vi "LoggerHelper-Pnumatics.vi"(8 "Stablizer":T1, 9 "Grabber":T1, 10 "Intake":T1, 11 "Shifter":T1) -> (2 "Logged PNU Output":string)   [LabVIEW 2014]
uses:
  <vilib>/Rock Robotics/WPI/Solenoid/WPI_SolenoidValue.ctl
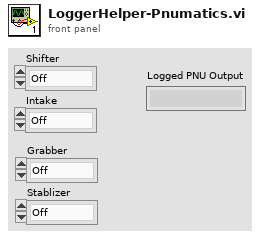
[diagram p1: front panel]
types:
  T1 = typedef "WPI_SolenoidValue.ctl" = enum16{"Off", "On", "Forward", "Reverse"}
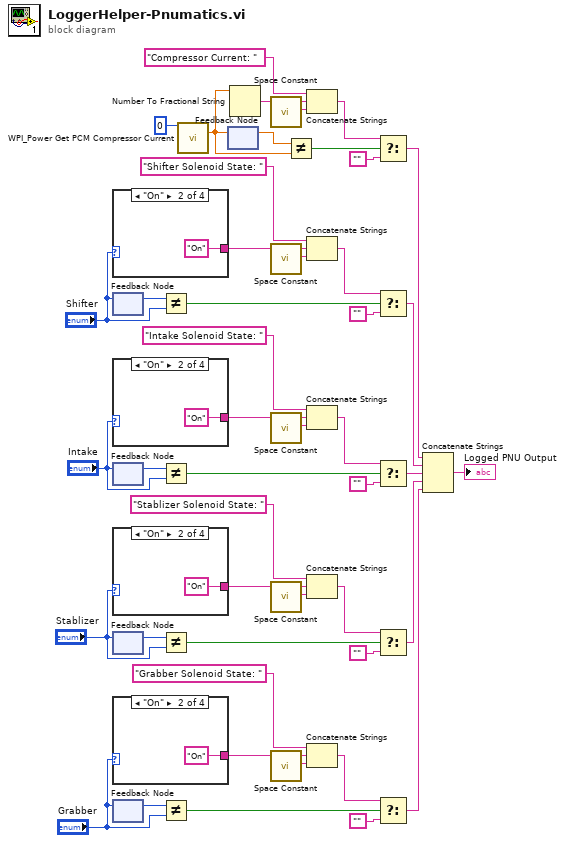
[diagram p0: block diagram]
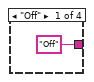
[diagram p2: hidden frame]
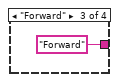
[diagram p3: hidden frame]
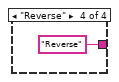
[diagram p4: hidden frame]
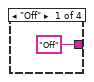
[diagram p5: hidden frame]
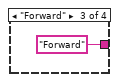
[diagram p6: hidden frame]
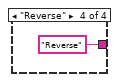
[diagram p7: hidden frame]
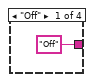
[diagram p8: hidden frame]
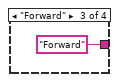
[diagram p9: hidden frame]
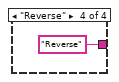
[diagram p10: hidden frame]
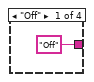
[diagram p11: hidden frame]
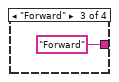
[diagram p12: hidden frame]
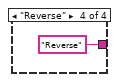
[diagram p13: hidden frame]
diagram:
  n1 = case shown="\"On\"" "Shifter" {
    tunnel: ["Off" "On" "Forward" "Reverse"] -> w24
    frame "Off" {
    }
    frame "On" {
    }
    frame "Forward" {
    }
    frame "Reverse" {
    }
  }
  n2 = feedback #1() -> (w42:T1)  [unwired: 1 in]
  n3 = feedback-in #1("Shifter") -> ()
  n4 = case shown="\"On\"" "Intake" {
    tunnel: ["Off" "On" "Forward" "Reverse"] -> w26
    frame "Off" {
    }
    frame "On" {
    }
    frame "Forward" {
    }
    frame "Reverse" {
    }
  }
  n5 = feedback #2() -> (w38:T1)  [unwired: 1 in]
  n6 = feedback-in #2("Intake") -> ()
  n7 = case shown="\"On\"" "Stablizer" {
    tunnel: ["Off" "On" "Forward" "Reverse"] -> w14
    frame "Off" {
    }
    frame "On" {
    }
    frame "Forward" {
    }
    frame "Reverse" {
    }
  }
  n8 = feedback #3() -> (w18:T1)  [unwired: 1 in]
  n9 = feedback-in #3("Stablizer") -> ()
  n10 = case shown="\"On\"" "Grabber" {
    tunnel: ["Off" "On" "Forward" "Reverse"] -> w8
    frame "Off" {
    }
    frame "On" {
    }
    frame "Forward" {
    }
    frame "Reverse" {
    }
  }
  n11 = feedback #4() -> (w12:T1)  [unwired: 1 in]
  n12 = feedback-in #4("Grabber") -> ()
  n13 = Not Equal?(x=w42, y="Shifter") -> (x != y?=w39:bool)
  n14 = Not Equal?(x=w38, y="Intake") -> (x != y?=w36:bool)
  n15 = Not Equal?(x=w18, y="Stablizer") -> (x != y?=w16:bool)
  n16 = Not Equal?(x=w12, y="Grabber") -> (x != y?=w10:bool)
  n17 = call <vilib>:"WPI_Power Get PCM Compressor Current.vi"("Pneumatics Control Module (0)"=u8 0) -> ("current (A)"=w43:dbl)  [unwired: 13 in, 1 out]
  n18 = feedback-in #5(w43) -> ()
  n19 = feedback #5() -> (w44:dbl)  [unwired: 1 in]
  n20 = Number To Fractional String(number=w43) -> (F-format string=w34:string)  [unwired: 3 in]
  n21 = call <vilib>:"Space Constant.vi"() -> ("String"=w30:string)
  n22 = call <vilib>:"Space Constant.vi"() -> ("String"=w29:string)
  n23 = call <vilib>:"Space Constant.vi"() -> ("String"=w28:string)
  n24 = call <vilib>:"Space Constant.vi"() -> ("String"=w15:string)
  n25 = call <vilib>:"Space Constant.vi"() -> ("String"=w9:string)
  n26 = Not Equal?(x=w44, y=w43) -> (x != y?=w46:bool)
  n27 = Concatenate Strings("Compressor Current: " ("string"), w34, w30) -> (w33:string)
  n28 = Concatenate Strings("Shifter Solenoid State: " ("string"), w24, w29) -> (w23:string)
  n29 = Concatenate Strings("Intake Solenoid State: " ("string"), w26, w28) -> (w25:string)
  n30 = Concatenate Strings("Stablizer Solenoid State: " ("string"), w14, w15) -> (w13:string)
  n31 = Concatenate Strings("Grabber Solenoid State: " ("string"), w8, w9) -> (w7:string)
  n32 = Select(t=w33, s=w46, f="") -> (s? t:f=w31:string)
  n33 = Select(t=w23, s=w39, f="") -> (s? t:f=w21:string)
  n34 = Select(t=w25, s=w36, f="") -> (s? t:f=w20:string)
  n35 = Select(t=w13, s=w16, f="") -> (s? t:f=w5:string)
  n36 = Select(t=w7, s=w10, f="") -> (s? t:f=w4:string)
  n37 = Concatenate Strings(w31, w21, w20, w5, w4) -> (→"Logged PNU Output":string)
